vi "UserDeletedRow Event Callback.vi"(4 "DataGridView in":refnum<class "DataGridView.lvclass">, 5 "Event Data":cluster{"sender":refnum<k24>, "e":refnum<k24>}, 6 "Control Ref":refnum<k24>, 7 "Event Common Data":T1) -> ()   [LabVIEW 2020, in "DataGrid.lvlib" / "DataGridView.lvclass"]
doc: "This callback fires when a row has been deleted from the datagrid, and will return the row"
uses:
  DataGridView/DataGridView.lvclass
  System.Windows.Forms
  UserDeletedRow/UserDeletedRow.lvclass
  C:/GEECS/Developers Version/source/Shared/LabVIEWdotNetDataGrid-master/source/Events/Abstract EVENT/Abstract EVENT.lvclass
  UserDeletedRow/UserDeletedRow.lvclass/UserDeletedRow.ctl
  UserDeletedRow/Write Row.vi
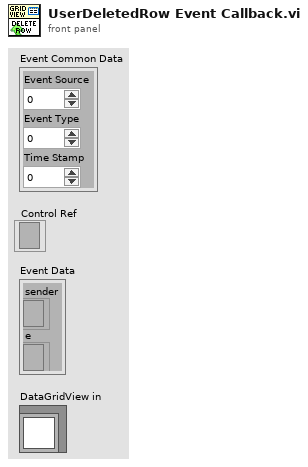
[diagram p1: front panel]
types:
  T1 = cluster{"Event Source":i32, "Event Type":u32, "Time Stamp":u32}
  T2 = cluster{"CellClicked":refnum<user-event>, "CellValue Changed":refnum<user-event>, "KeyDown":refnum<user-event>, "DataError":refnum<user-event>, "UserAddedRow":refnum<user-event>, "UserDeletedRow":refnum<user-event>, "CellDirtyStateChanged":refnum<user-event>}
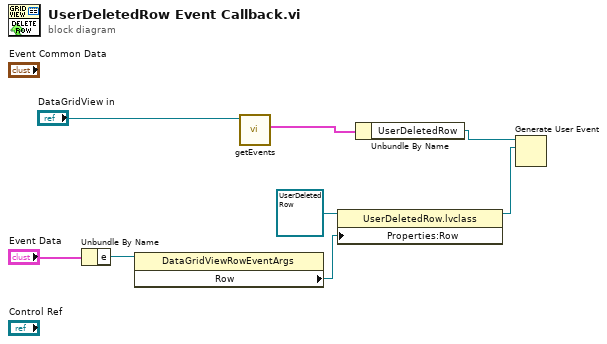
[diagram p0: block diagram]
diagram:
  n1 = Unbundle By Name("Event Data") -> ("e"=w6:refnum<k24>)
  n2 = property class="DataGridViewRowEventArgs"(reference=w6) -> ("Row"=w5:refnum<k24>)  [unwired: 1 in, 2 out]
  n3 = call "getEvents.vi"("DataGridView in"="DataGridView in") -> ("userEvents"=w8:T2)  [unwired: 8 in, 2 out]
  n4 = property class="UserDeletedRow.lvclass"(reference=refnum<class "UserDeletedRow.lvclass"> refnum ("DataGrid.lvlib:UserDeletedRow.lvclass"), "Properties:Row"=w5) -> (reference out=w4:refnum<class "UserDeletedRow.lvclass">)  [unwired: 1 in, 1 out]
  n5 = Unbundle By Name(w8) -> ("UserDeletedRow"=w7:refnum<user-event>)
  n6 = Generate User Event(user event=w7, event data cluster=w4) -> ()  [unwired: 2 in, 2 out]
